vi "waitTarget-Y.vi"(0 "Device in X":refnum<k24>, 5 "GetPOS X":refnum<vi>, 7 "Position X":sgl, 9 "GetPOS Y":refnum<vi>, 11 "Device in Y":refnum<k24>, 12 "Position Y":sgl) -> (4 "Device out X":refnum<k24>, 6 "GetPOS X":dbl format="%#_6f", 8 "GetPOS Y":dbl format="%#_6f", 15 "Device out Y":refnum<k24>)   [LabVIEW 2014]
doc: "André Romero - 2018\nandretec@ifsc.usp.br"
uses:
  C:/user-Lab/AndreTec/GITs/andretec/Thorlabs-Vector-Move/kinesisTec/Kinesis/Thorlabs.MotionControl.TCube.DCServoCLI.dll
  kinesisTec/Kinesis/Thorlabs.MotionControl.TCube.DCServoCLI.dll
panel:
  in  "error":dbl=0.004 format="%#_13g"
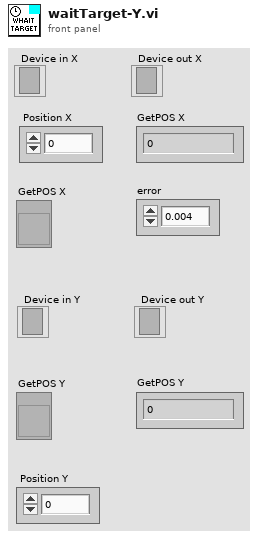
[diagram p1: front panel]
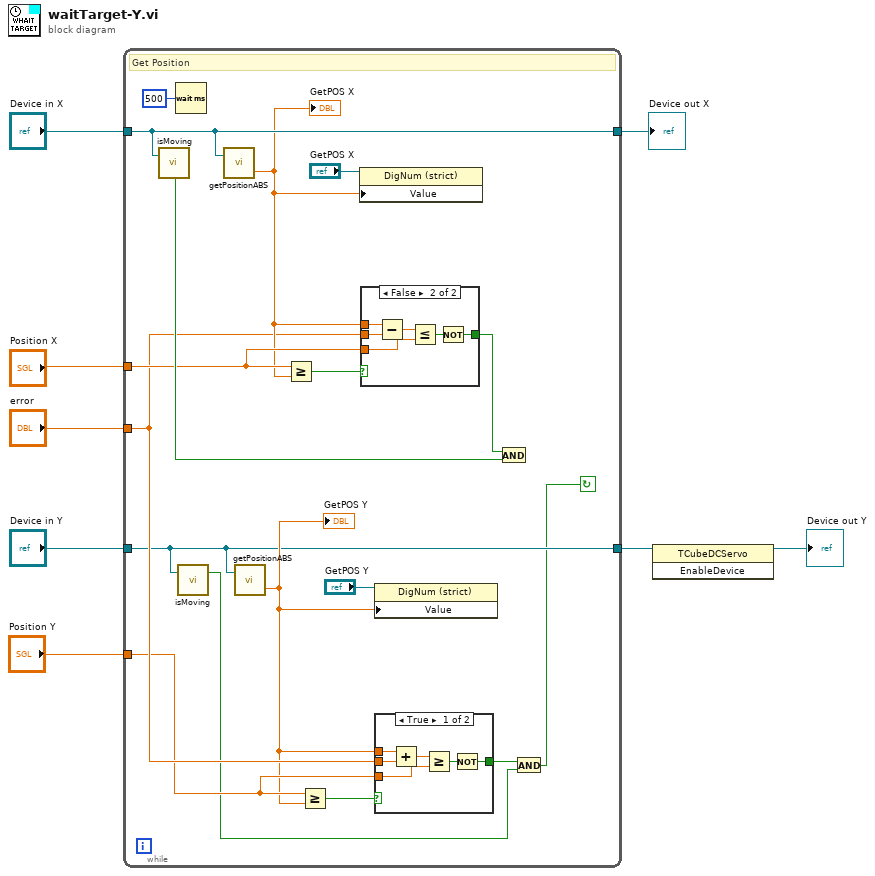
[diagram p0: block diagram]
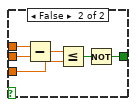
[diagram p2: hidden frame]
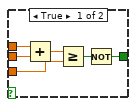
[diagram p3: hidden frame]
diagram:
  n1 = while {
    tunnel: "Device in X" -> [w25]
    tunnel: [w25] -> w7
    tunnel: "Position X" -> [w20]
    tunnel: "error" -> [w15]
    tunnel: "Device in Y" -> [w11]
    tunnel: [w11] -> w3
    tunnel: "Position Y" -> [w14]
    stop <- w9 continue-if-true
    # "Get Position"
    n2 = call "isMoving.vi"("Device in"=w25) -> ("IsMoving"=w23:bool)  [unwired: 1 in, 1 out]
    n3 = Wait (ms)(milliseconds to wait=u32 500) -> ()  [unwired: 1 out]
    n4 = call "isMoving.vi"("Device in"=w11) -> ("IsMoving"=w10:bool)  [unwired: 1 in, 1 out]
    n5 = call "getPositionABS.vi"("Device"=w25) -> ("GetPOS"=w18:dbl)  [unwired: 1 in, 1 out]
    "GetPOS X" <- w18
    n6 = call "getPositionABS.vi"("Device"=w11) -> ("GetPOS"=w12:dbl)  [unwired: 1 in, 1 out]
    "GetPOS Y" <- w12
    n7 = Greater Or Equal?(x=w20, y=w18) -> (x >= y?=w21:bool)
    n8 = Greater Or Equal?(x=w14, y=w12) -> (x >= y?=w16:bool)
    n9 = property class="DigNum (strict)"(reference="GetPOS X", "Value"=w18) -> ()  [unwired: 1 in, 2 out]
    n10 = case shown="False" w21 {
      tunnel: w18 -> [w43 w49]
      tunnel: w15 -> [w42 w48]
      tunnel: w20 -> [w40 w46]
      tunnel: [w38 w44] -> w19
      frame True {
        n11 = Add(x=w43, y=w42) -> (x+y=w41:dbl)
        n12 = Greater Or Equal?(x=w41, y=w40) -> (x >= y?=w39:bool)
        n13 = Not(x=w39) -> (.not. x?=w38:bool)
      }
      frame False {
        n14 = Subtract(x=w49, y=w48) -> (x-y=w47:dbl)
        n15 = Less Or Equal?(x=w47, y=w46) -> (x <= y?=w45:bool)
        n16 = Not(x=w45) -> (.not. x?=w44:bool)
      }
    }
    n17 = property class="DigNum (strict)"(reference="GetPOS Y", "Value"=w12) -> ()  [unwired: 1 in, 2 out]
    n18 = case shown="True" w16 {
      tunnel: w12 -> [w31 w37]
      tunnel: w15 -> [w30 w36]
      tunnel: w14 -> [w28 w34]
      tunnel: [w26 w32] -> w13
      frame True {
        n19 = Add(x=w31, y=w30) -> (x+y=w29:dbl)
        n20 = Greater Or Equal?(x=w29, y=w28) -> (x >= y?=w27:bool)
        n21 = Not(x=w27) -> (.not. x?=w26:bool)
      }
      frame False {
        n22 = Subtract(x=w37, y=w36) -> (x-y=w35:dbl)
        n23 = Less Or Equal?(x=w35, y=w34) -> (x <= y?=w33:bool)
        n24 = Not(x=w33) -> (.not. x?=w32:bool)
      }
    }
    n25 = And(x=w19, y=w23) -> ()  [unwired: 1 out]
    n26 = And(x=w13, y=w10) -> (x .and. y?=w9:bool)
  }
  "Device out X" <- w7
  n27 = invoke class="TCubeDCServo" method="EnableDevice"(reference=w3) -> (reference out=→"Device out Y":refnum<k24>)  [unwired: 2 in, 2 out]
